vi "PreBuildTest(Pass).vi"(8 "error in (no error)":errorcluster) -> (0 "error out":errorcluster)   [LabVIEW 2020]
uses:
  classes/Test Suite/Test Suite.lvclass
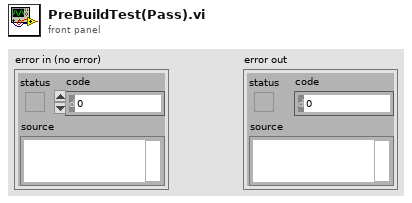
[diagram p1: front panel]
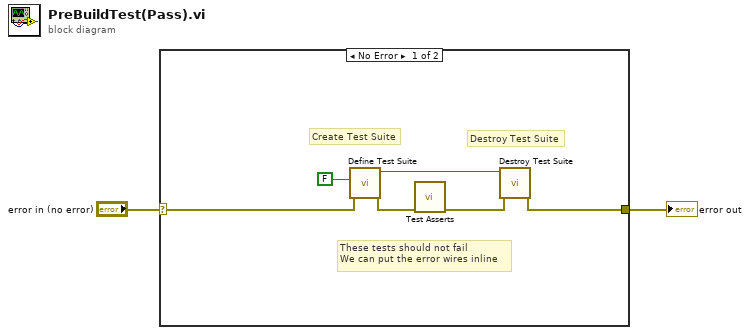
[diagram p0: block diagram]
diagram:
  n1 = case shown="No Error" "error in (no error)" {
    selector: "error in (no error)" -> [w7 w9]
    tunnel: [w3 w9] -> w2
    frame No Error {
      # "Destroy Test Suite"
      # "Create Test Suite"
      # "These tests should not fail\nWe can put the error wires inline"
      n2 = call "Define Test Suite.vi"("error in (no error)"=w7, "Interactive"=FALSE) -> ("error out"=w6:errorcluster, "Test Suite"=w5:refnum<class "Test Suite.lvclass">)  [unwired: 7 in, 1 out]
      n3 = call "Test Asserts.vi"("error in (no error)"=w6) -> ("error out"=w4:errorcluster)  [unwired: 10 in]
      n4 = call-dynamic "Destroy Test Suite.vi"("error in (no error)"=w4, "Test Suite in"=w5) -> ("error out"=w3:errorcluster)  [unwired: 8 in, 1 out]
    }
    frame Error {
    }
  }
  "error out" <- w2
